vi "Seriennummer ermitteln.vi"(8 "error in (no error)":errorcluster caption="Fehler (Eingang, kein Fehler)", 10 "Istwerte":u16[](array[numeric]), 11 "Steuerung PNS Eingang":refnum<class "Steuerung PNS.lvclass">) -> (0 "error out":errorcluster caption="Fehler (Ausgang)", 2 "Seriennummer":string, 3 "Steuerung PNS Ausgang":refnum<class "Steuerung PNS.lvclass">)   [LabVIEW 2020, in "Steuerung PNS.lvclass"]
uses:
  Steuerung PNS.lvclass
  Steuerung PNS.lvclass/Steuerung PNS.ctl
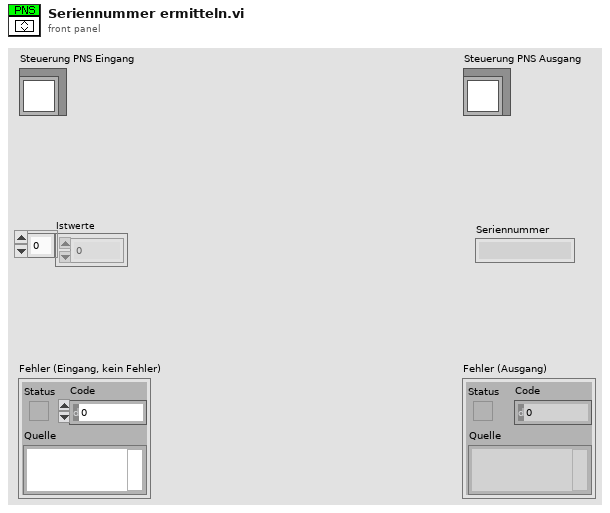
[diagram p1: front panel]
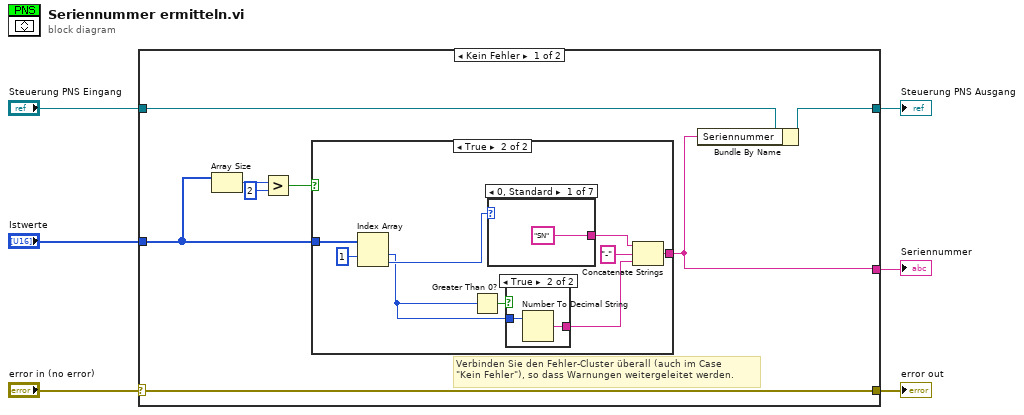
[diagram p0: block diagram]
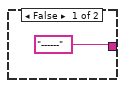
[diagram p2: hidden frame]
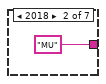
[diagram p4: hidden frame]
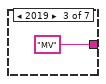
[diagram p5: hidden frame]
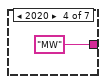
[diagram p6: hidden frame]
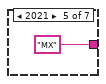
[diagram p7: hidden frame]
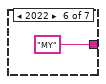
[diagram p8: hidden frame]
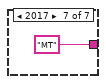
[diagram p9: hidden frame]
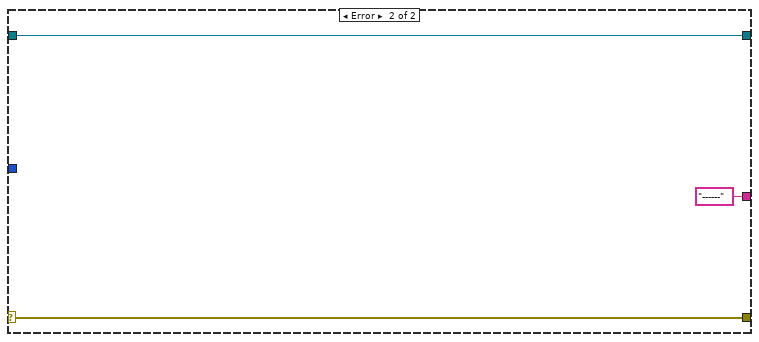
[diagram p10: hidden frame]
diagram:
  n1 = case shown="Kein Fehler" "error in (no error)" {
    selector: "error in (no error)" -> [w14 w36]
    tunnel: [w14 w36] -> w5
    tunnel: [w12 w35] -> w3
    tunnel: "Steuerung PNS Eingang" -> [w13 w35]
    tunnel: "Istwerte" -> [w10 _]
    tunnel: [w11 "------"] -> w1
    frame No Error {
      # "Verbinden Sie den Fehler-Cluster überall (auch im Case\n\"Kein Fehler\"), so dass Warnungen weitergeleitet werden."
      n2 = Array Size(array=w10) -> (size(s)=w9:i32)
      n3 = Greater?(x=w9, y=2) -> (0:w7:bool)
      n4 = case shown="True" w7 {
        tunnel: ["------" w20] -> w11
        tunnel: w10 -> [_ w19]
        frame False {
        }
        frame True {
          n5 = Index Array(array=w19, index #1=1 ("Index")) -> (element #1=w17:u16, element #2=w23:u16)  [unwired: 1 in]
          n6 = Greater Than 0?(x=w17) -> (x > 0?=w16:bool)
          n7 = case shown="0, Standard" w23 {
            tunnel: ["SN" "MU" "MV" "MW" "MX" "MY" "MT"] -> w22
            frame 0, Default {
            }
            frame 2018 {
            }
            frame 2019 {
            }
            frame 2020 {
            }
            frame 2021 {
            }
            frame 2022 {
            }
            frame 2017 {
            }
          }
          n8 = case shown="True" w16 {
            tunnel: w17 -> [_ w26]
            tunnel: [_ w25] -> w18
            frame False {
            }
            frame True {
              n9 = Number To Decimal String(number=w26) -> (decimal integer string=w25:string)  [unwired: 1 in]
            }
          }
          n10 = Concatenate Strings(w22, "-", w18) -> (w20:string)
        }
      }
      n11 = Bundle By Name(cluster=w13, "Seriennummer"=w11) -> (w12:refnum<class "Steuerung PNS.lvclass">)
    }
    frame Error {
    }
  }
  "error out" <- w5
  "Steuerung PNS Ausgang" <- w3
  "Seriennummer" <- w1
